vi "GOMDBTS2048 calib Wavelength Measure Lamp.vi"(8 "error in (no error)":errorcluster, 10 "lampnumber":i32, 11 "handle":i32) -> (0 "error out":errorcluster, 2 "function return":i32)   [LabVIEW 2015, in "GOMDBTS2048.lvlib"]
doc: "GOBTS2048DLL int __stdcall GOMDBTS2048_calibGetFilterAssignment(int handle, int* value);"
uses:
  GOMDBTS2048.lvlib
  runtime/GOMDBTS2048.dll
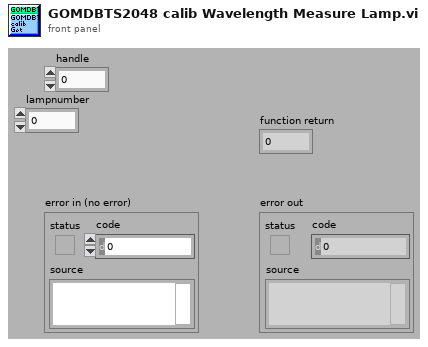
[diagram p1: front panel]
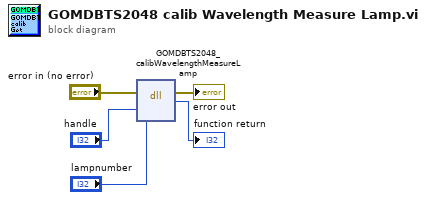
[diagram p0: block diagram]
diagram:
  n1 = dll-call lib="C:/Users/rkoch/Documents/GO_Library/runtime/GOMDBTS2048.*" fn="GOMDBTS2048_calibWavelengthMeasureLamp"(error in="error in (no error)", "handle"="handle", "lampnumber"="lampnumber") -> (error out=→"error out":errorcluster, "return type"=→"function return":i32)  [unwired: 4 in, 1 out]
